vi "Tx_Create FIFO Param Disable Association.vi"(8 "error in (no error)":errorcluster, 11 "Input Channel Data []":T4[](array[typedef]) {"Labels Settings"."Word"."Param Setting"."Num Bits" min=1 max=32; "Labels Settings"."Word"."Param Setting"."Start Bit" min=8 max=31}) -> (0 "error out":errorcluster, 2 "Raw Values":T1, 3 "Map":T3[](array[typedef]))   [LabVIEW 2017, in "Ballard Arinc-429 Engine.lvlib"]
doc: "This VI creates a static association between NI-VS FIFO Channel Index and Physical Channel, Label Index, Parameter Index and whether it's a parameter channel or a disable channel."
uses:
  Ballard Arinc-429 Engine.lvlib
  RT Controls/RT HW Channel.ctl
  RT Controls/RT Label Settings.ctl
  Shared/Controls and Global/Label.ctl
  Shared/Controls and Global/transferPeriod.ctl
  RT Controls/RT Word Settings.ctl
  RT Controls/RT Param Setting.ctl
  Shared/Controls and Global/Start Bit.ctl
  Shared/Controls and Global/Number of Bits.ctl
  Shared/Controls and Global/TransferType.ctl
  RT Controls/RT Tx Association.ctl
  RT Controls/RT Tx Default Raw Value.ctl
  RT Controls/RT Tx Default Raw Value_Association.ctl
  Shared/Ballard Arinc-429 Shared.lvlib
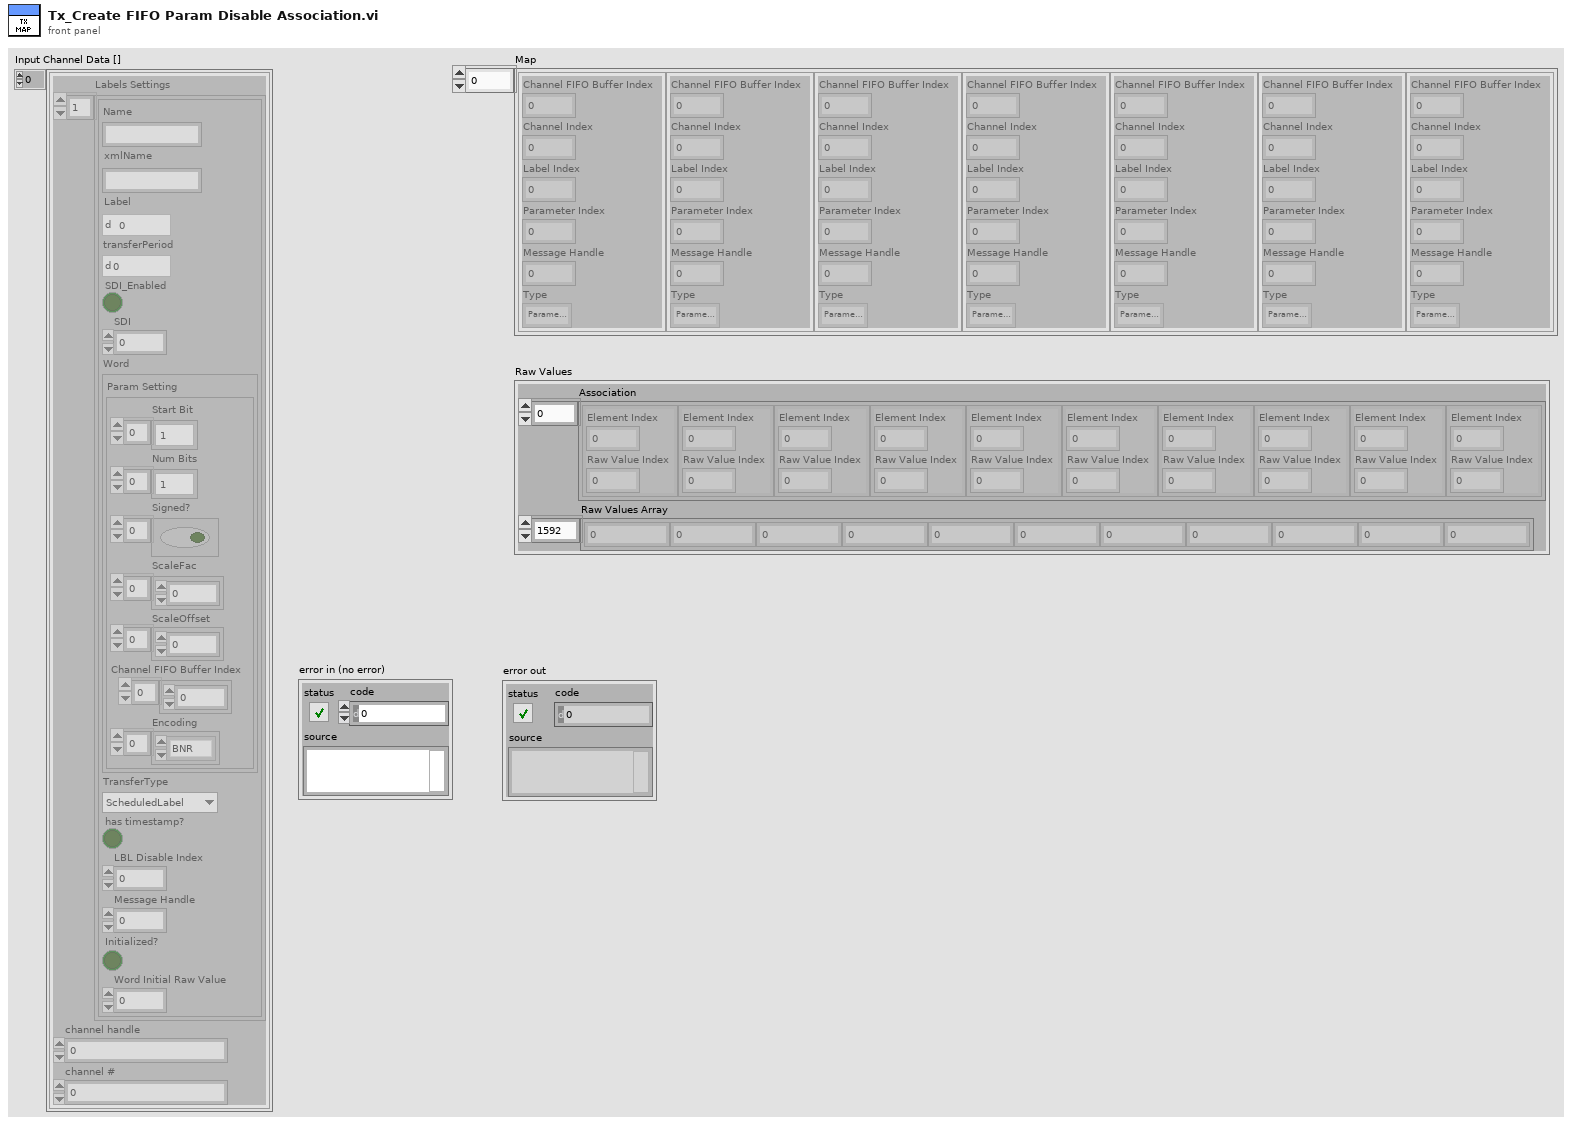
[diagram p1: front panel]
types:
  T1 = typedef "Ballard Arinc-429 Engine.lvlib/RT Tx Default Raw Value.ctl" = cluster{"Association":T2[], "Raw Values Array":u32[]}
  T2 = typedef "Ballard Arinc-429 Engine.lvlib/RT Tx Default Raw Value_Association.ctl" = cluster{"Element Index":i32, "Raw Value Index":i32}
  T3 = typedef "Ballard Arinc-429 Engine.lvlib/RT Tx Association.ctl" = cluster{"Channel FIFO Buffer Index":i32, "Channel Index":i32, "Label Index":i32, "Parameter Index":i32, "Message Handle":u64, "Type":enum16{"Parameter Channel", "Disable Channel"}}
  T4 = typedef "Ballard Arinc-429 Engine.lvlib/RT HW Channel.ctl" = cluster{"Labels Settings":T5[], "channel handle":u32, "channel #":u16}
  T5 = typedef "Ballard Arinc-429 Engine.lvlib/RT Label Settings.ctl" = cluster{"Name":string, "xmlName":string, "Label":T6, "transferPeriod":T7, "SDI_Enabled":bool, "SDI":u8, "Word":T8, "TransferType":T12, "has timestamp?":bool, "LBL Disable Index":i32, "Message Handle":u64, "Initialized?":bool, "Word Initial Raw Value":u32}
  T6 = typedef "Ballard Arinc-429 Shared.lvlib/Label.ctl" = u8
  T7 = typedef "Ballard Arinc-429 Shared.lvlib/transferPeriod.ctl" = u32
  T8 = typedef "Ballard Arinc-429 Engine.lvlib/RT Word Settings.ctl" = cluster{"Param Setting":T9}
  T9 = typedef "Ballard Arinc-429 Engine.lvlib/RT Param Setting.ctl" = cluster{"Start Bit":T10[], "Num Bits":T11[], "Signed?":bool[], "ScaleFac":dbl[], "ScaleOffset":dbl[], "Channel FIFO Buffer Index":i32[], "Encoding":enum16{"BNR", "BCD", "Discrete"}[]}
  T10 = typedef "Ballard Arinc-429 Shared.lvlib/Start Bit.ctl" = i32
  T11 = typedef "Ballard Arinc-429 Shared.lvlib/Number of Bits.ctl" = i32
  T12 = typedef "Ballard Arinc-429 Shared.lvlib/TransferType.ctl" = enum16{"ScheduledLabel", "Acyclic", "Block", "Strobe"}
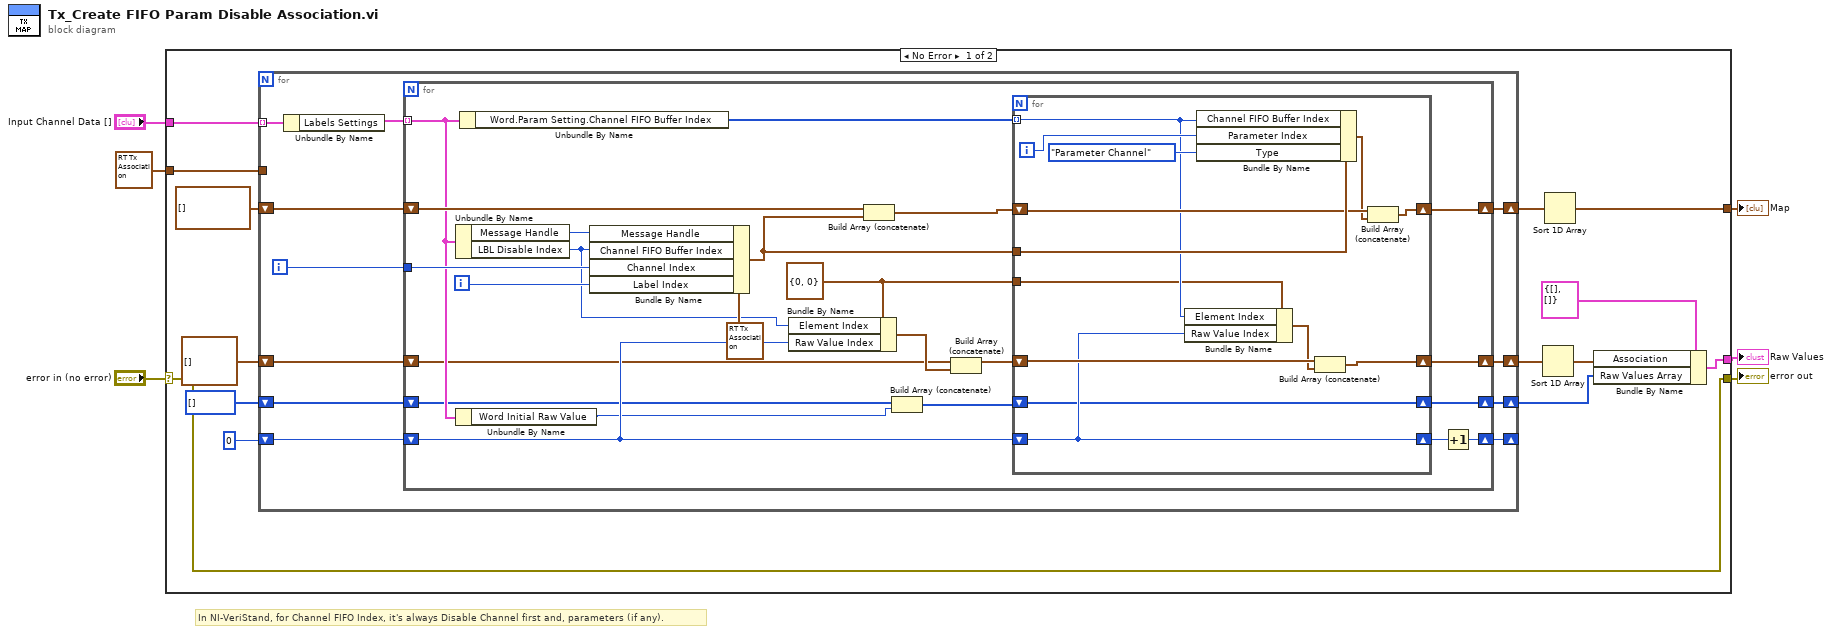
[diagram p0: block diagram]
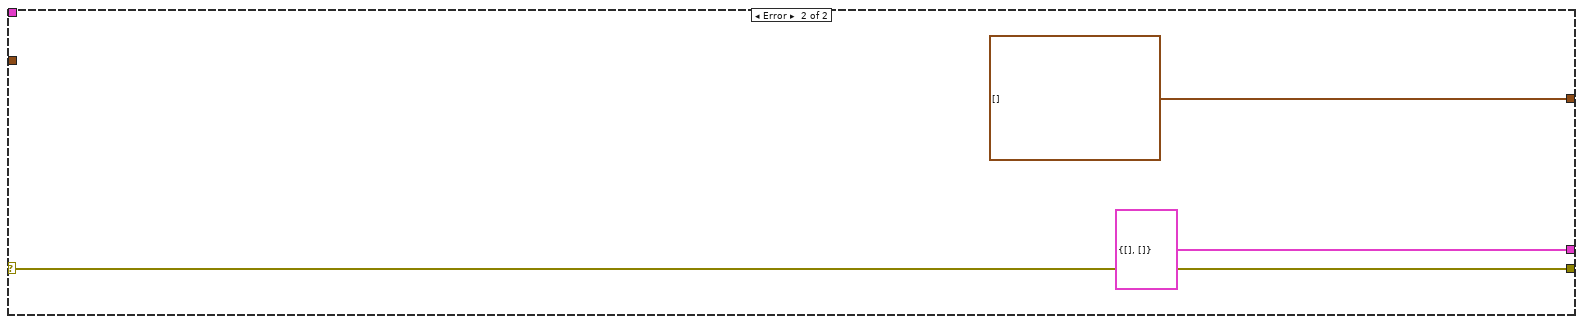
[diagram p2: hidden frame]
diagram:
  # "In NI-VeriStand, for Channel FIFO Index, it's always Disable Channel first and, parameters (if any)."
  n1 = case shown="No Error" "error in (no error)" {
    selector: "error in (no error)" -> [w17 w70]
    tunnel: [w17 w70] -> w5
    tunnel: "Input Channel Data []" -> [w20 _]
    tunnel: T3 {"Channel FIFO Buffer Index"=0, "Channel Index"=0, "Label Index"=0, "Parameter Index"=0, "Message Handle"=0, "Type"=enum."Parameter Channel"} ("Association") -> [w19 _]
    tunnel: [w15 T3[] []] -> w2
    tunnel: [w10 T1 {"Association"=[], "Raw Values Array"=[]}] -> w1
    frame No Error {
      n2 = for {
        tunnel: w20 -> [w30] mode=indexing
        tunnel: w19 -> [_]
        shift-right: [w27] -> w16
        shift-left: T3[] [] -> [w29]
        shift-right: [w25] -> w13
        shift-left: T2[] [] -> [w26]
        shift-right: [w21] -> w8
        shift-left: u32[] [] -> [w24]
        shift-right: [w22] -> _
        shift-left: 0 -> [w23]
        i -> [w28]
        n3 = Unbundle By Name(w30) -> ("Labels Settings"=w31:T5[])
        n4 = for {
          tunnel: w31 -> [w44] mode=indexing
          shift-right: [w49] -> w27
          shift-left: w29 -> [w51]
          tunnel: w28 -> [w52]
          shift-right: [w45] -> w25
          shift-left: w26 -> [w37]
          shift-right: [w43] -> w21
          shift-left: w24 -> [w35]
          shift-right: [w41] -> w22
          shift-left: w23 -> [w40]
          i -> [w46]
          w39 = T2 {"Element Index"=0, "Raw Value Index"=0}
          n5 = Unbundle By Name(w44) -> ("Message Handle"=w53:u64, "LBL Disable Index"=w32:i32)
          n6 = Unbundle By Name(w44) -> ("Word Initial Raw Value"=w34:u32)
          n7 = Unbundle By Name(w44) -> ("Word.Param Setting.Channel FIFO Buffer Index"=w47:i32[])
          n8 = Bundle By Name(cluster=T3 {"Channel FIFO Buffer Index"=0, "Channel Index"=0, "Label Index"=0, "Parameter Index"=-1, "Message Handle"=0, "Type"=enum."Disable Channel"} ("Association"), "Message Handle"=w53, "Channel FIFO Buffer Index"=w32, "Channel Index"=w52, "Label Index"=w46) -> (w48:T3)
          n9 = Bundle By Name(cluster=w39, "Element Index"=w32, "Raw Value Index"=w40) -> (w38:T2)
          n10 = Build Array (concatenate)(w51, w48) -> (w50:T3[])
          n11 = Build Array (concatenate)(w35, w34) -> (w33:u32[])
          n12 = Build Array (concatenate)(w37, w38) -> (w36:T2[])
          n13 = for {
            shift-right: [w63] -> w49
            shift-left: w50 -> [w65]
            tunnel: w48 -> [w67]
            tunnel: w47 -> [w58] mode=indexing
            shift-right: [w60] -> w45
            shift-left: w36 -> [w61]
            shift-right: [w55] -> w43
            shift-left: w33 -> [w55]
            shift-right: [w59] -> w42
            shift-left: w40 -> [w59]
            tunnel: w39 -> [w56]
            i -> [w62]
            n14 = Bundle By Name(cluster=w56, "Element Index"=w58, "Raw Value Index"=w59) -> (w57:T2)
            n15 = Bundle By Name(cluster=w67, "Channel FIFO Buffer Index"=w58, "Parameter Index"=w62, "Type"=enum16{"Parameter Channel", "Disable Channel"}."Parameter Channel") -> (w64:T3)
            n16 = Build Array (concatenate)(w61, w57) -> (w60:T2[])
            n17 = Build Array (concatenate)(w65, w64) -> (w63:T3[])
          }
          n18 = Increment(x=w42) -> (x+1=w41:i32)
        }
      }
      n19 = Sort 1D Array(array=w13) -> (sorted array=w11:T2[])
      n20 = Sort 1D Array(array=w16) -> (sorted array=w15:T3[])
      n21 = Bundle By Name(cluster=T1 {"Association"=[], "Raw Values Array"=[]} ("Raw Values"), "Association"=w11, "Raw Values Array"=w8) -> (w10:T1)
    }
    frame Error {
    }
  }
  "error out" <- w5
  "Map" <- w2
  "Raw Values" <- w1
